vi "325 Read and Compressor auto control(SubVI).vi"(11 "Instrument":T2={"335 Resource"="", "Input (0:A)"=0, "Instrument Type"=enum."PPMS", "quantum design"=refnum, "Heater Output (1:1)"=0, "semaphore"=refnum, "TCP master instance"=refnum, "335 Status"=refnum, "M24C Resource"="GPIB0::24::INSTR", "4G supply"="GPIB0::24::INSTR", "Temp Status 24C"=refnum, "Temp"=refnum, "9T信号"=refnum, "limit"={"Field limit"=0.0, "Field rate limit"=0.0, "Temp limit"=0.0, "Temp low limit"=0.0, "Temp rate limit "=0.0}, "4g supply status"=refnum, "vi路径"="", "325 Resource "="GPIB0::24::INSTR", "Input (0:A) 325"=0, "Input (1;B)"=1, "in-plane"="", "out-plane"="", "in-plane"=FALSE, "out-plane"=FALSE, "in plane 信号"=refnum, "pzt volt"=refnum, "Aborting"=refnum, "数据文件"=refnum, "warning"=refnum, "750 visa"="", "750 rotate"="", "335 Status 2"=refnum} {"Input (1;B)" items=["A", "B"]; "Input (0:A) 325" items=["A", "B"]; "Input (0:A)" items=["A", "B"]; "Heater Output (1:1)" items=["1"=1, "2"=2]}) -> (2 "325 Temp":dbl, 3 "簇":T6 {"Heater Range" items=["Off", "Low (On)", "Medium", "High"]; "Heater Range 2" items=["Off", "Low (On)", "Medium", "High"]; "?" items=["Unknow", "Stable", "Following Warm", "Following Cold", "Unfollowing"]})   [LabVIEW 2019, in "Get value.lvlib"]
uses:
  Get value.lvlib
  ctl/335 state.ctl
  ctl/Instrument.ctl
  <vilib>/NI/Modbus Library/API/Master/Modbus Master.lvclass
  ctl/Instrument Type.ctl
  lib/QDInstrument.dll
  ctl/limit.ctl
  ctl/9T mag field stauts.ctl
  ctl/warning.ctl
  lib/Lake Shore 335/Lake Shore 335.lvlib
panel:
  out "下拉列表":T1=2 items=["Unknow", "Stable", "Following Warm", "Following Cold", "Unfollowing"]
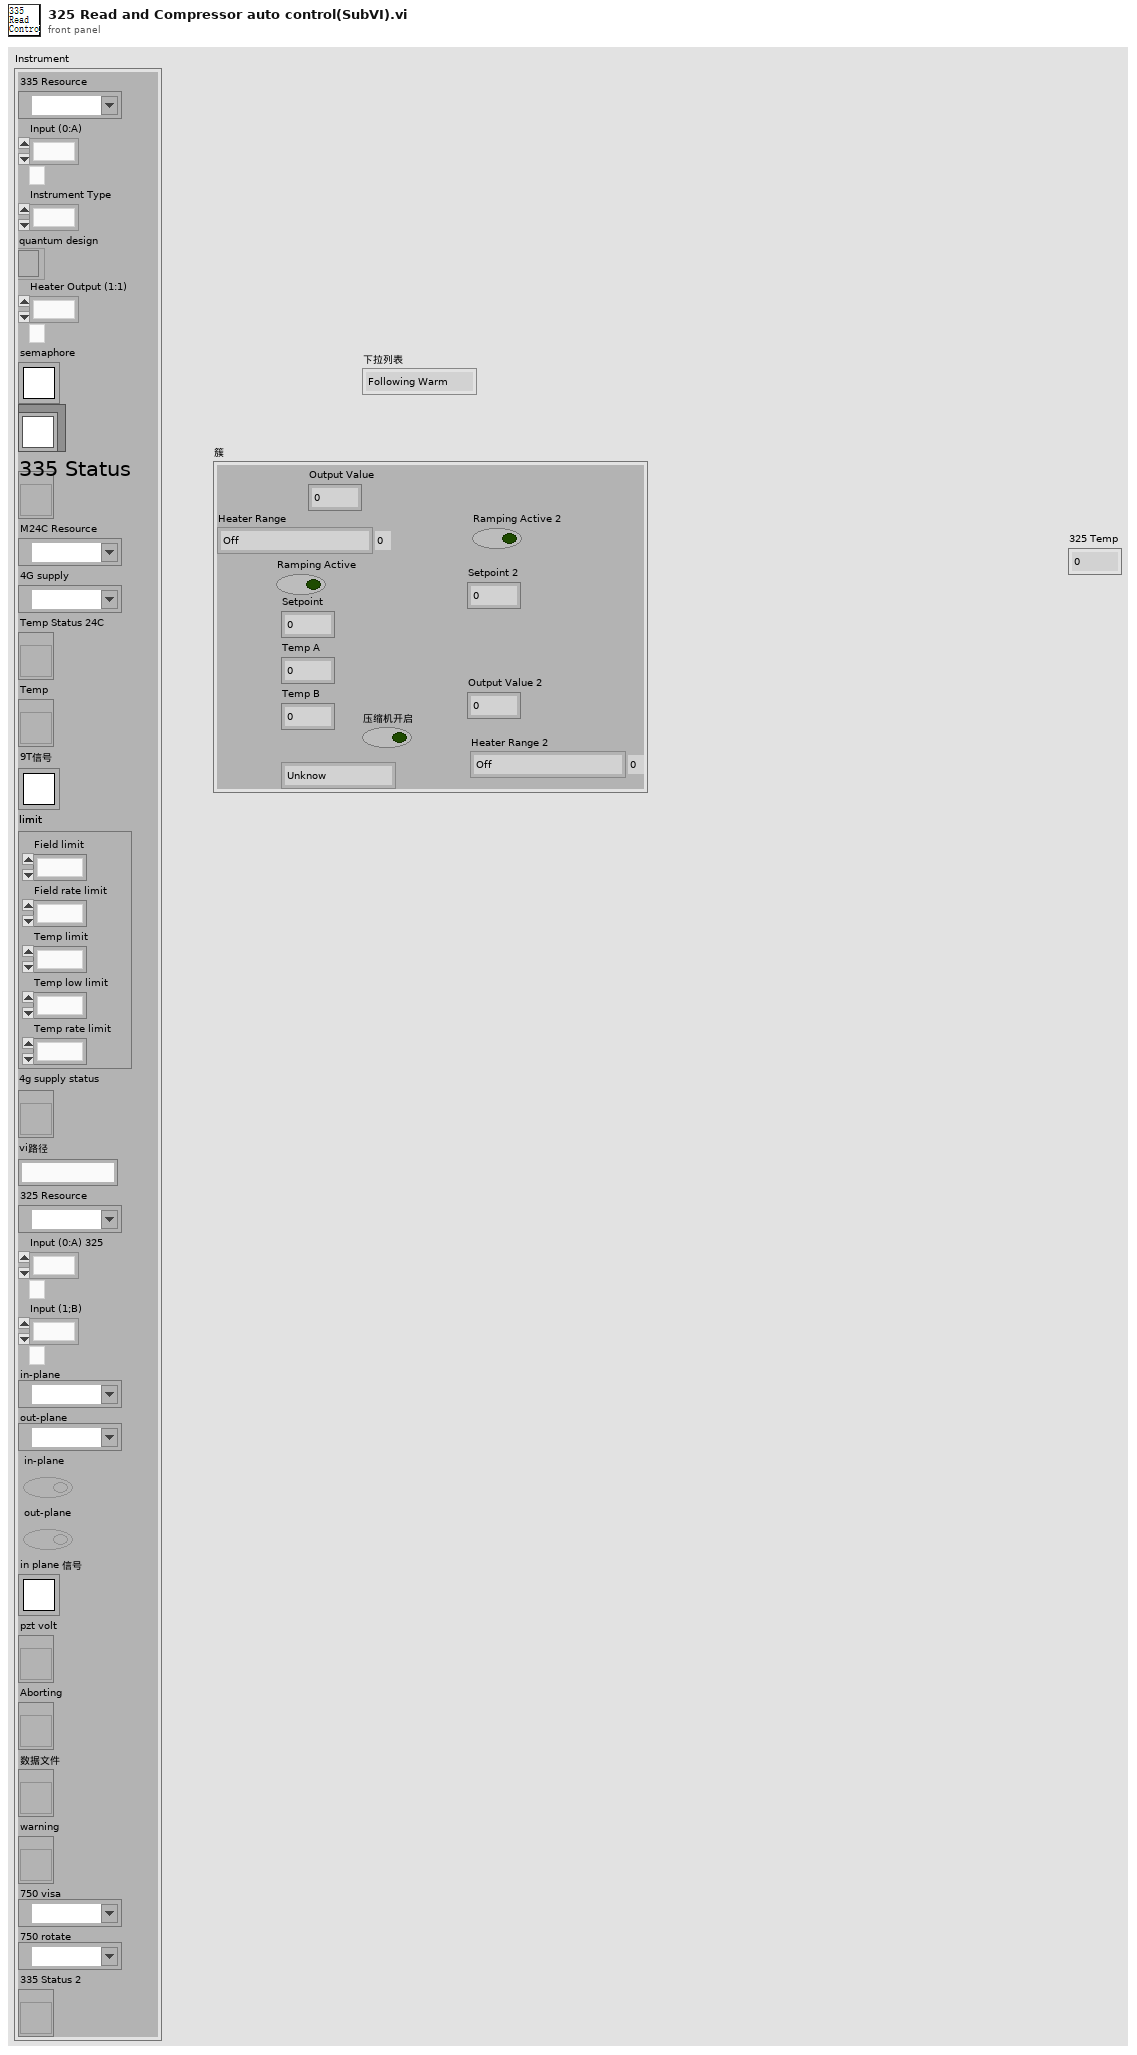
[diagram p1: front panel]
types:
  T1 = typedef "335 state.ctl" = u16
  T2 = typedef "Instrument.ctl" = cluster{"335 Resource":refnum<visa-resource-name>, "Input (0:A)":u16, "Instrument Type":T3, "quantum design":refnum<k24>, "Heater Output (1:1)":u16, "semaphore":T4, "TCP master instance":refnum<class "Modbus Master.lvclass">, "335 Status":refnum<vi>, "M24C Resource":refnum<visa-resource-name>, "4G supply":refnum<visa-resource-name>, "Temp Status 24C":refnum<vi>, "Temp":refnum<vi>, "9T信号":T4, "limit":T5, "4g supply status":refnum<vi>, "vi路径":string, "325 Resource ":refnum<visa-resource-name>, "Input (0:A) 325":u16, "Input (1;B)":u16, "in-plane":refnum<visa-resource-name>, "out-plane":refnum<visa-resource-name>, "in-plane":bool, "out-plane":bool, "in plane 信号":T4, "pzt volt":refnum<vi>, "Aborting":refnum<vi>, "数据文件":refnum<vi>, "warning":refnum<vi>, "750 visa":refnum<visa-resource-name>, "750 rotate":refnum<visa-resource-name>, "335 Status 2":refnum<vi>}
  T3 = typedef "Instrument Type.ctl" = enum16{"PPMS", "VersaLab", "DynaCool", "SVSM", "PPMS-Rotate", "Lakeshore335", "lengtou2", "9T mag", "9T cmag rotate", "test"}
  T4 = typedef "Semaphore RefNum" = refnum<k1>
  T5 = typedef "limit.ctl" = cluster{"Field limit":dbl, "Field rate limit":dbl, "Temp limit":dbl, "Temp low limit":dbl, "Temp rate limit ":dbl}
  T6 = cluster{"Output Value":dbl, "Heater Range":u16, "Ramping Active":bool, "Setpoint":dbl, "Temp A":dbl, "Temp B":dbl, "压缩机开启":bool, T1, "Ramping Active 2":bool, "Setpoint 2":dbl, "Output Value 2":dbl, "Heater Range 2":u16}
  T7 = cluster{"Output Value":dbl, "Heater Range ":u16, "Ramping Active":bool, "Setpoint":dbl, "Sensor Data":dbl, "Sensor Data":dbl, bool, T1, "Ramping Active":bool, "Setpoint":dbl, "Output Value":dbl, "Heater Range ":u16}
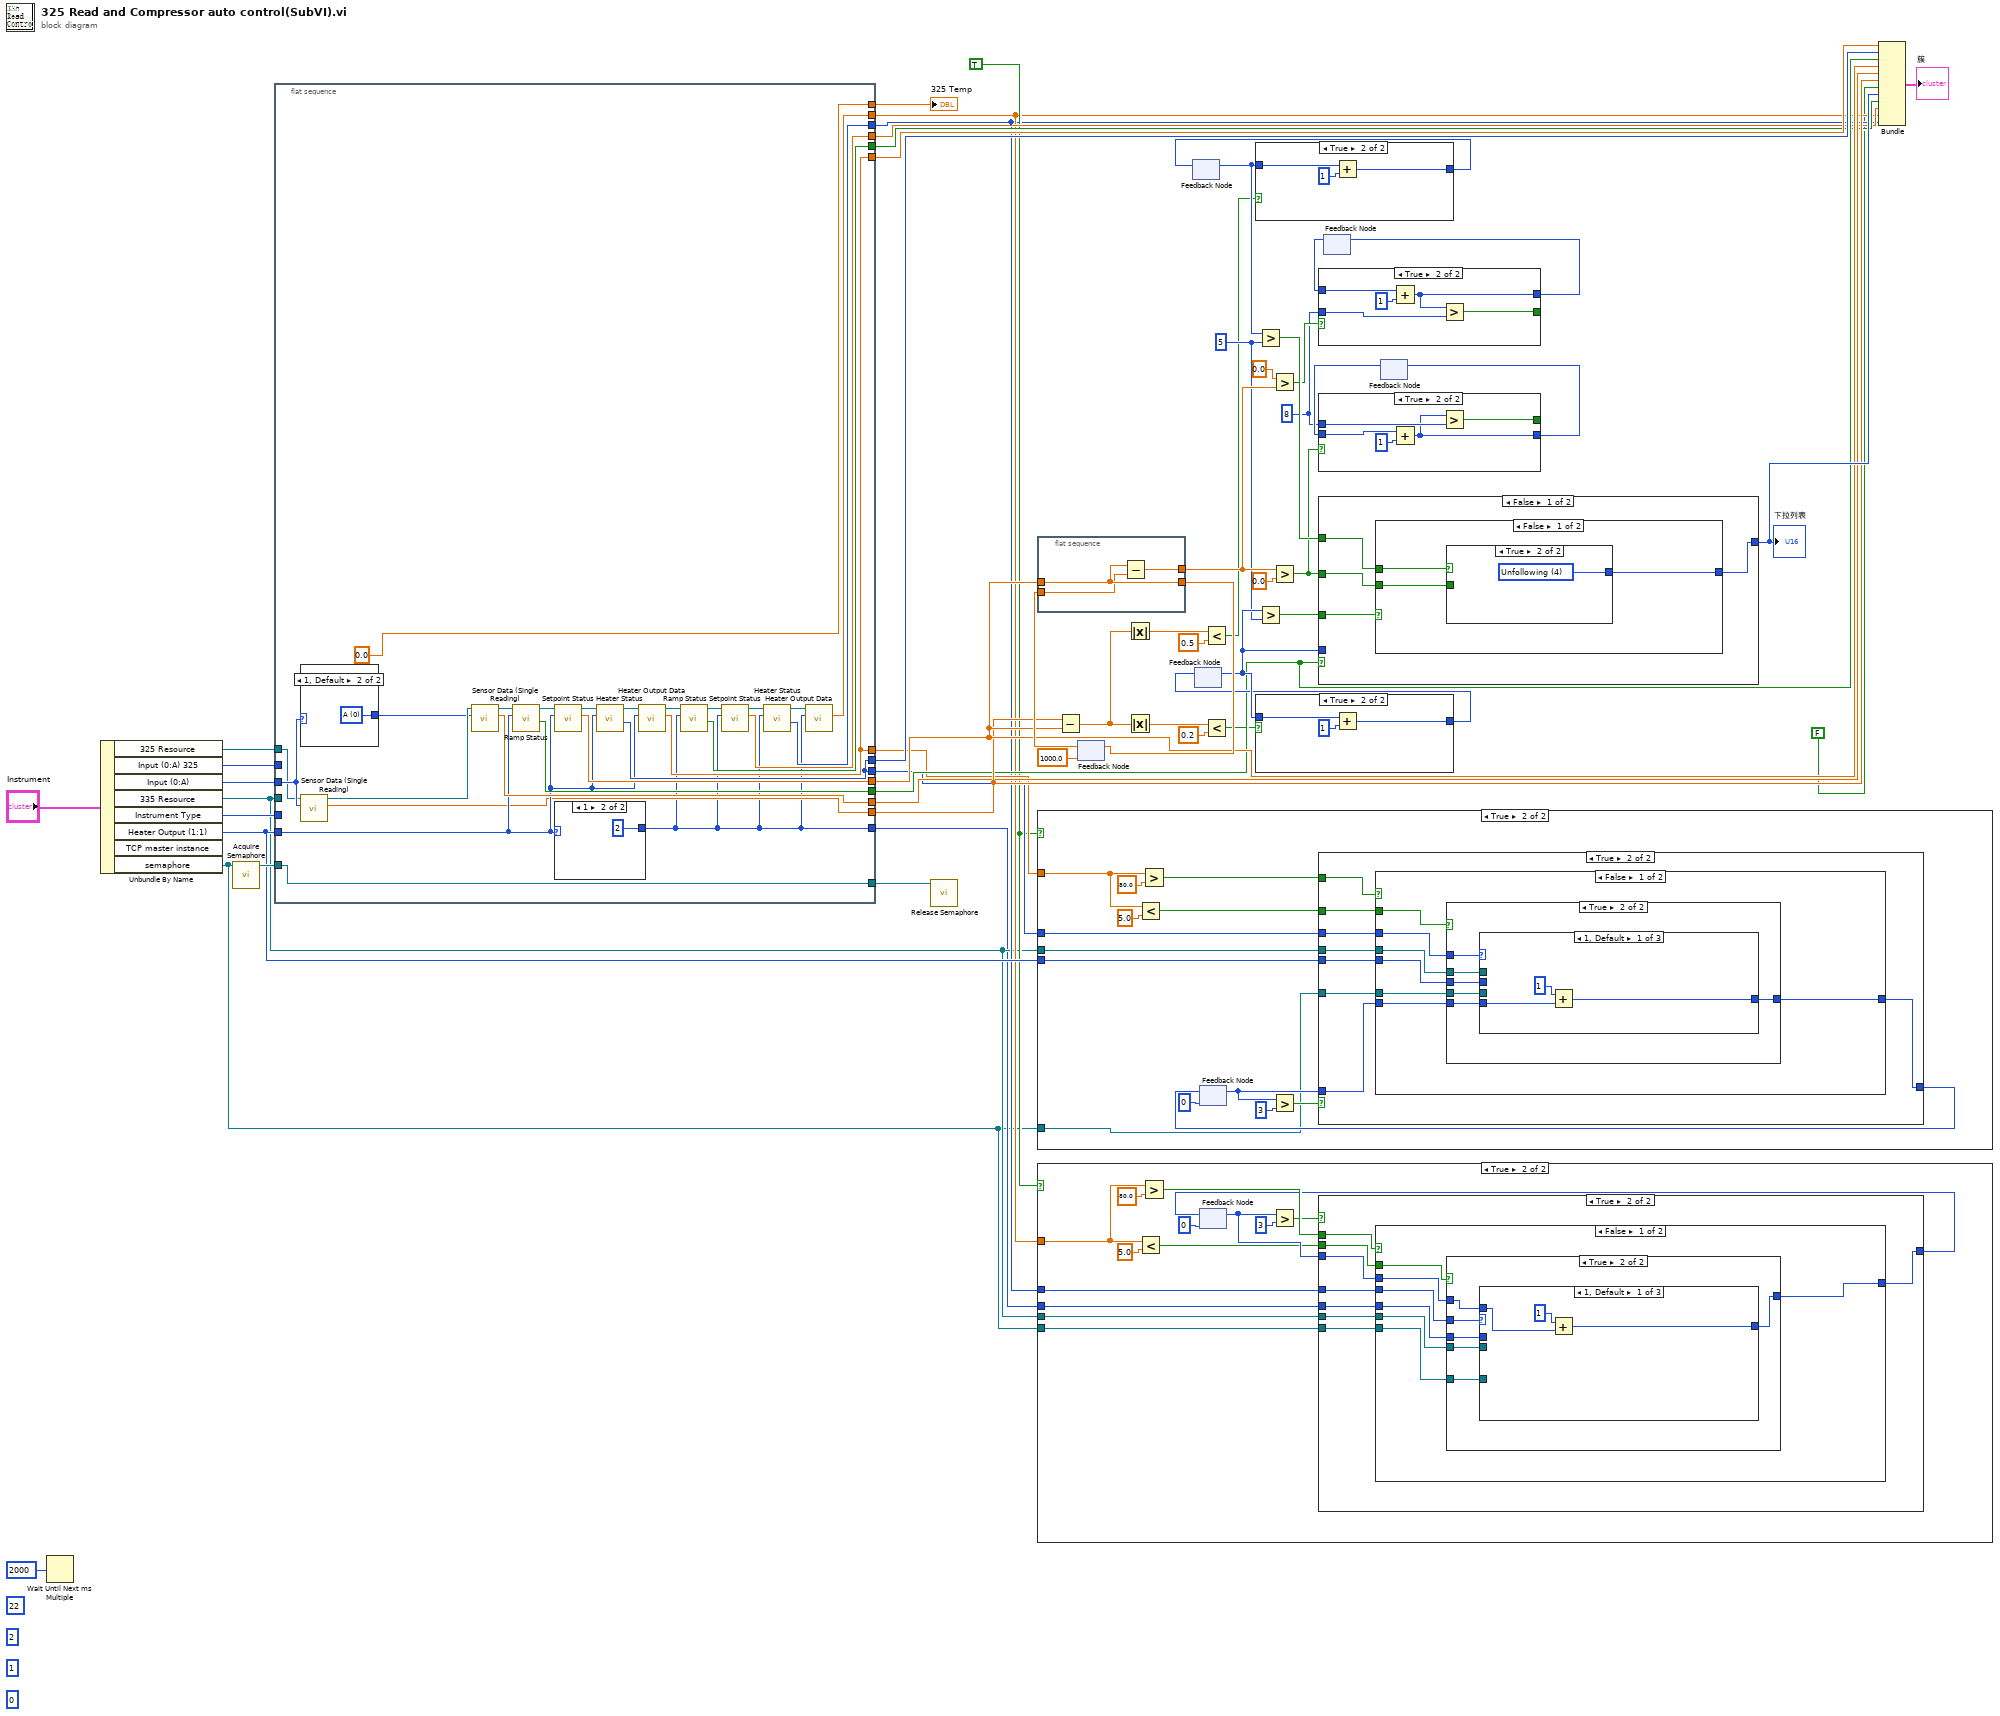
[diagram p0: block diagram]
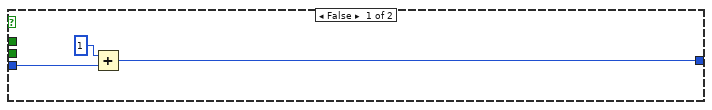
[diagram p3: hidden frame]
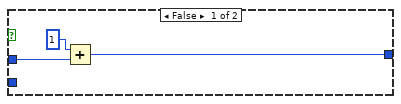
[diagram p4: hidden frame]
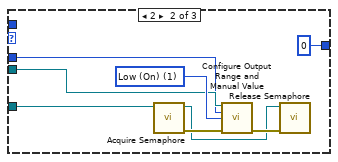
[diagram p5: hidden frame]
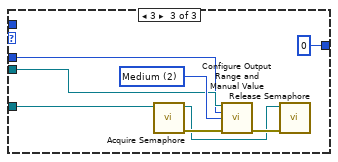
[diagram p6: hidden frame]
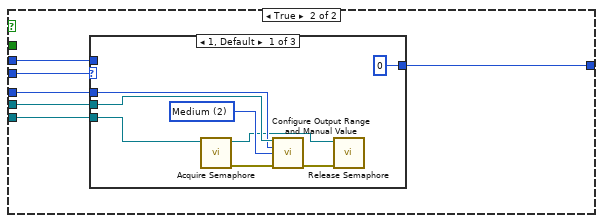
[diagram p7: hidden frame]
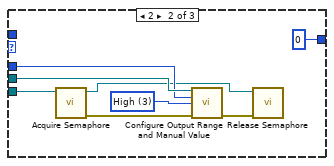
[diagram p8: hidden frame]
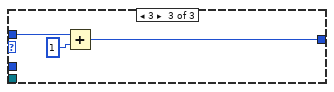
[diagram p9: hidden frame]
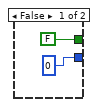
[diagram p10: hidden frame]
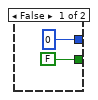
[diagram p11: hidden frame]
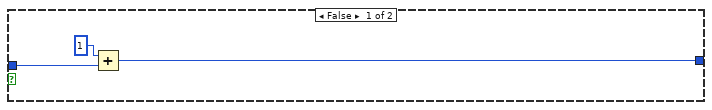
[diagram p13: hidden frame]
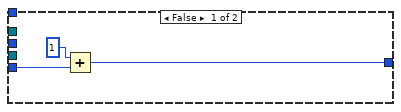
[diagram p14: hidden frame]
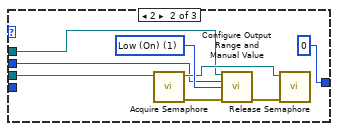
[diagram p15: hidden frame]
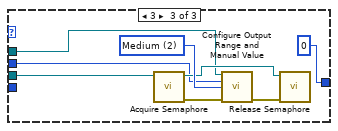
[diagram p16: hidden frame]
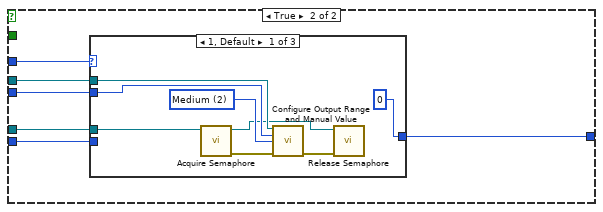
[diagram p17: hidden frame]
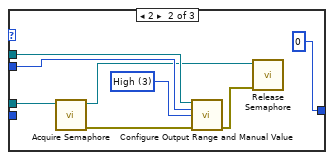
[diagram p18: hidden frame]
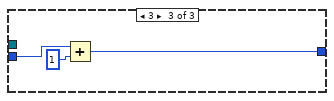
[diagram p19: hidden frame]
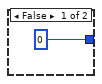
[diagram p20: hidden frame]
diagram:
  w14 = 8 ("y")
  w8 = TRUE
  w40 = 5 ("y")
  (unwired) 1 ("index")
  (unwired) 0 ("index")
  (unwired) u16 2 ("number of inputs")
  (unwired) u16 22 ("starting address")
  n1 = Wait Until Next ms Multiple(millisecond multiple=u32 2000) -> ()  [unwired: 1 out]
  n2 = Unbundle By Name("Instrument") -> ("325 Resource"=w13:refnum<visa-resource-name>, "Input (0:A) 325"=w12:u16, "Input (0:A)"=w28:u16, "335 Resource"=w5:refnum<visa-resource-name>, "Instrument Type"=w25:T3, "Heater Output (1:1)"=w21:u16, "semaphore"=w3:T4)  [unwired: 1 out]
  n3 = call <vilib>:"Acquire Semaphore.vi"("semaphore"=w3) -> ("semaphore out"=w26:T4)  [unwired: 4 in, 2 out]
  n4 = flat-sequence {
    tunnel: [w82] -> w49
    tunnel: w5 -> [_]
    tunnel: [w61] -> w44
    tunnel: w25 -> [_]
    tunnel: w26 -> [w78]
    tunnel: [w78] -> w27
    tunnel: [w72] -> w30
    tunnel: [w73] -> w29
    tunnel: [w77] -> w43
    tunnel: w21 -> [w66]
    tunnel: w28 -> [w60]
    tunnel: [w74] -> w31
    tunnel: [w73] -> w23
    tunnel: [w72] -> w22
    tunnel: w13 -> [w57]
    tunnel: w12 -> [_]
    tunnel: [0.0 ("Sensor Data")] -> w11
    tunnel: [w65] -> w10
    tunnel: [w64] -> w9
    tunnel: [w63] -> w6
    tunnel: [w62] -> w7
    tunnel: [w59] -> w4
    frame #0 {
      n5 = case shown="1, Default" w60 {
        tunnel: [w85 w86] -> w71
        frame 0 {
          w85 = u16 1 items=["A", "B"] ("Input (0:A)")
        }
        frame 1, Default {
          w86 = u16 0 items=["A", "B"] ("Input (0:A)")
        }
      }
      n6 = call "Sensor Data (Single Reading).vi"("Input (0:A)"=w60, "VISA resource name"=w57) -> ("Sensor Data"=w61:dbl, "VISA resource name out"=w76:refnum<visa-resource-name>)  [unwired: 7 in, 1 out]
      n7 = call "Sensor Data (Single Reading).vi"("Input (0:A)"=w71, "VISA resource name"=w76) -> ("Sensor Data"=w74:dbl, "VISA resource name out"=w75:refnum<visa-resource-name>)  [unwired: 7 in, 1 out]
      n8 = call "Ramp Status.vi"("Output's Control Loop (1:1)"=w66, "VISA resource name"=w75) -> ("Ramping Active"=w77:bool, "VISA resource name out"=w81:refnum<visa-resource-name>)  [unwired: 5 in, 3 out]
      n9 = call "Setpoint Status.vi"("Output (1:1)"=w66, "VISA resource name"=w81) -> ("Setpoint"=w82:dbl, "VISA resource name out"=w80:refnum<visa-resource-name>)  [unwired: 7 in, 1 out]
      n10 = case shown="1" w66 {
        tunnel: [1 2] -> w59
        frame 2, Default {
        }
        frame 1 {
        }
      }
      n11 = call "Heater Status.vi"("Heater Output (1:1)"=w66, "VISA resource name"=w80) -> ("Heater Range"=w72:u16, "VISA resource name out"=w79:refnum<visa-resource-name>)  [unwired: 5 in, 3 out]
      n12 = call "Heater Output Data.vi"("Heater Output (1:1)"=w66, "VISA resource name"=w79) -> ("Output Value"=w73:dbl, "VISA resource name out"=w70:refnum<visa-resource-name>)  [unwired: 7 in, 1 out]
      n13 = call "Ramp Status.vi"("Output's Control Loop (1:1)"=w59, "VISA resource name"=w70) -> ("Ramping Active"=w65:bool, "VISA resource name out"=w69:refnum<visa-resource-name>)  [unwired: 5 in, 3 out]
      n14 = call "Setpoint Status.vi"("Output (1:1)"=w59, "VISA resource name"=w69) -> ("Setpoint"=w64:dbl, "VISA resource name out"=w68:refnum<visa-resource-name>)  [unwired: 7 in, 1 out]
      n15 = call "Heater Status.vi"("Heater Output (1:1)"=w59, "VISA resource name"=w68) -> ("Heater Range"=w63:u16, "VISA resource name out"=w67:refnum<visa-resource-name>)  [unwired: 5 in, 3 out]
      n16 = call "Heater Output Data.vi"("Heater Output (1:1)"=w59, "VISA resource name"=w67) -> ("Output Value"=w62:dbl)  [unwired: 7 in, 2 out]
    }
  }
  n17 = call <vilib>:"Release Semaphore.vi"("semaphore"=w27) -> ()  [unwired: 5 in, 2 out]
  n18 = flat-sequence {
    tunnel: w49 -> [w89]
    tunnel: [w89] -> w50
    tunnel: w51 -> [w88]
    tunnel: [w87] -> w56
    frame #0 {
      n19 = Subtract(x=w89, y=w88) -> (x-y=w87:dbl)
    }
  }
  n20 = case shown="True" w8 {
    tunnel: w23 -> [_ w102]
    tunnel: w22 -> [_ w99]
    tunnel: w5 -> [_ w98]
    tunnel: w21 -> [_ w97]
    tunnel: w3 -> [_ w90]
    frame False {
    }
    frame True {
      n21 = Less?(x=w102, y=5.0) -> (x < y?=w92:bool)
      n22 = Greater?(x=w102, y=80.0) -> (0:w100:bool)
      n23 = feedback #1(0) -> (w93:i32)
      n24 = Greater?(x=w93, y=3) -> (0:w95:bool)
      n25 = case shown="True" w95 {
        tunnel: w100 -> [_ w114]
        tunnel: w99 -> [_ w113]
        tunnel: w98 -> [_ w112]
        tunnel: w97 -> [_ w111]
        tunnel: w90 -> [_ w110]
        tunnel: [w104 w109] -> w94
        tunnel: w93 -> [w106 w108]
        tunnel: w92 -> [_ w107]
        frame False {
          n26 = Add(x=1, y=w106) -> (x+y=w104:i32)
        }
        frame True {
          n27 = case shown="False" w114 {
            tunnel: w113 -> [w121 w155]
            tunnel: w112 -> [w120 w154]
            tunnel: w111 -> [w119 w153]
            tunnel: w110 -> [w116 w152]
            tunnel: [w118 w151] -> w109
            tunnel: w108 -> [w117 w150]
            tunnel: w107 -> [w115 _]
            frame False {
              n28 = case shown="True" w115 {
                tunnel: w121 -> [_ w130]
                tunnel: w120 -> [_ w129]
                tunnel: w119 -> [_ w128]
                tunnel: [w122 w127] -> w118
                tunnel: w117 -> [w124 w126]
                tunnel: w116 -> [_ w125]
                frame False {
                  n29 = Add(x=1, y=w124) -> (x+y=w122:i32)
                }
                frame True {
                  n30 = case shown="1, Default" w130 {
                    tunnel: w129 -> [_ w137 w145]
                    tunnel: w128 -> [_ w136 w144]
                    tunnel: [w131 0 0] -> w127
                    tunnel: w126 -> [w133 _ _]
                    tunnel: w125 -> [_ w134 w142]
                    frame 1, Default {
                      n31 = Add(x=1, y=w133) -> (x+y=w131:i32)
                    }
                    frame 2 {
                      w141 = u16 1 items=["Off", "Low (On)", "Medium", "High"] ("Range (0:Off)")
                      n32 = call <vilib>:"Acquire Semaphore.vi"("semaphore"=w134) -> ("error out"=w140:errorcluster, "semaphore out"=w138:T4)  [unwired: 4 in, 1 out]
                      n33 = call "Configure Output Range and Manual Value.vi"("VISA resource name"=w137, "Heater Output (1:1)"=w136, "Range (0:Off)"=w141, "error in (no error)"=w140) -> ("error out"=w139:errorcluster)  [unwired: 10 in, 1 out]
                      n34 = call <vilib>:"Release Semaphore.vi"("error in (no error)"=w139, "semaphore"=w138) -> ()  [unwired: 4 in, 2 out]
                    }
                    frame 3 {
                      w149 = u16 2 items=["Off", "Low (On)", "Medium", "High"] ("Range (0:Off)")
                      n35 = call <vilib>:"Acquire Semaphore.vi"("semaphore"=w142) -> ("error out"=w148:errorcluster, "semaphore out"=w146:T4)  [unwired: 4 in, 1 out]
                      n36 = call "Configure Output Range and Manual Value.vi"("VISA resource name"=w145, "Heater Output (1:1)"=w144, "Range (0:Off)"=w149, "error in (no error)"=w148) -> ("error out"=w147:errorcluster)  [unwired: 10 in, 1 out]
                      n37 = call <vilib>:"Release Semaphore.vi"("error in (no error)"=w147, "semaphore"=w146) -> ()  [unwired: 4 in, 2 out]
                    }
                  }
                }
              }
            }
            frame True {
              n38 = case shown="1, Default" w155 {
                tunnel: w154 -> [w163 w171 _]
                tunnel: w153 -> [w162 w170 _]
                tunnel: w152 -> [w156 w165 _]
                tunnel: [0 0 w172] -> w151
                tunnel: w150 -> [_ _ w174]
                frame 1, Default {
                  w159 = u16 2 items=["Off", "Low (On)", "Medium", "High"] ("Range (0:Off)")
                  n39 = call <vilib>:"Acquire Semaphore.vi"("semaphore"=w156) -> ("error out"=w160:errorcluster, "semaphore out"=w158:T4)  [unwired: 4 in, 1 out]
                  n40 = call "Configure Output Range and Manual Value.vi"("VISA resource name"=w163, "Heater Output (1:1)"=w162, "Range (0:Off)"=w159, "error in (no error)"=w160) -> ("error out"=w161:errorcluster)  [unwired: 10 in, 1 out]
                  n41 = call <vilib>:"Release Semaphore.vi"("error in (no error)"=w161, "semaphore"=w158) -> ()  [unwired: 4 in, 2 out]
                }
                frame 2 {
                  w169 = u16 3 items=["Off", "Low (On)", "Medium", "High"] ("Range (0:Off)")
                  n42 = call <vilib>:"Acquire Semaphore.vi"("semaphore"=w165) -> ("error out"=w168:errorcluster, "semaphore out"=w166:T4)  [unwired: 4 in, 1 out]
                  n43 = call "Configure Output Range and Manual Value.vi"("VISA resource name"=w171, "Heater Output (1:1)"=w170, "Range (0:Off)"=w169, "error in (no error)"=w168) -> ("error out"=w167:errorcluster)  [unwired: 10 in, 1 out]
                  n44 = call <vilib>:"Release Semaphore.vi"("error in (no error)"=w167, "semaphore"=w166) -> ()  [unwired: 4 in, 2 out]
                }
                frame 3 {
                  n45 = Add(x=w174, y=1) -> (x+y=w172:i32)
                }
              }
            }
          }
        }
      }
      n46 = feedback-in #1(w94) -> ()
    }
  }
  n47 = case shown="True" w8 {
    tunnel: w7 -> [_ w187]
    tunnel: w6 -> [_ w184]
    tunnel: w5 -> [_ w183]
    tunnel: w4 -> [_ w182]
    tunnel: w3 -> [_ w181]
    frame False {
    }
    frame True {
      n48 = Less?(x=w187, y=5.0) -> (x < y?=w176:bool)
      n49 = Greater?(x=w187, y=80.0) -> (0:w185:bool)
      n50 = feedback #2(0) -> (w177:i32)
      n51 = Greater?(x=w177, y=3) -> (0:w179:bool)
      n52 = case shown="True" w179 {
        tunnel: w185 -> [_ w199]
        tunnel: w184 -> [_ w198]
        tunnel: w183 -> [_ w197]
        tunnel: w182 -> [_ w196]
        tunnel: w181 -> [_ w195]
        tunnel: [w189 w194] -> w178
        tunnel: w177 -> [w191 w193]
        tunnel: w176 -> [_ w192]
        frame False {
          n53 = Add(x=1, y=w191) -> (x+y=w189:i32)
        }
        frame True {
          n54 = case shown="False" w199 {
            tunnel: w198 -> [w206 w240]
            tunnel: w197 -> [w205 w239]
            tunnel: w196 -> [w204 w238]
            tunnel: w195 -> [w201 w237]
            tunnel: [w203 w236] -> w194
            tunnel: w193 -> [w202 w235]
            tunnel: w192 -> [w200 _]
            frame False {
              n55 = case shown="True" w200 {
                tunnel: w206 -> [_ w215]
                tunnel: w205 -> [_ w214]
                tunnel: w204 -> [_ w213]
                tunnel: [w207 w212] -> w203
                tunnel: w202 -> [w209 w211]
                tunnel: w201 -> [_ w210]
                frame False {
                  n56 = Add(x=1, y=w209) -> (x+y=w207:i32)
                }
                frame True {
                  n57 = case shown="1, Default" w215 {
                    tunnel: w214 -> [_ w222 w230]
                    tunnel: w213 -> [_ w221 w229]
                    tunnel: [w216 0 0] -> w212
                    tunnel: w211 -> [w218 _ _]
                    tunnel: w210 -> [_ w219 w227]
                    frame 1, Default {
                      n58 = Add(x=1, y=w218) -> (x+y=w216:i32)
                    }
                    frame 2 {
                      w226 = u16 1 items=["Off", "Low (On)", "Medium", "High"] ("Range (0:Off)")
                      n59 = call <vilib>:"Acquire Semaphore.vi"("semaphore"=w219) -> ("error out"=w225:errorcluster, "semaphore out"=w223:T4)  [unwired: 4 in, 1 out]
                      n60 = call "Configure Output Range and Manual Value.vi"("VISA resource name"=w222, "Heater Output (1:1)"=w221, "Range (0:Off)"=w226, "error in (no error)"=w225) -> ("error out"=w224:errorcluster)  [unwired: 10 in, 1 out]
                      n61 = call <vilib>:"Release Semaphore.vi"("error in (no error)"=w224, "semaphore"=w223) -> ()  [unwired: 4 in, 2 out]
                    }
                    frame 3 {
                      w234 = u16 2 items=["Off", "Low (On)", "Medium", "High"] ("Range (0:Off)")
                      n62 = call <vilib>:"Acquire Semaphore.vi"("semaphore"=w227) -> ("error out"=w233:errorcluster, "semaphore out"=w231:T4)  [unwired: 4 in, 1 out]
                      n63 = call "Configure Output Range and Manual Value.vi"("VISA resource name"=w230, "Heater Output (1:1)"=w229, "Range (0:Off)"=w234, "error in (no error)"=w233) -> ("error out"=w232:errorcluster)  [unwired: 10 in, 1 out]
                      n64 = call <vilib>:"Release Semaphore.vi"("error in (no error)"=w232, "semaphore"=w231) -> ()  [unwired: 4 in, 2 out]
                    }
                  }
                }
              }
            }
            frame True {
              n65 = case shown="1, Default" w240 {
                tunnel: w239 -> [w248 w256 _]
                tunnel: w238 -> [w247 w255 _]
                tunnel: w237 -> [w241 w250 _]
                tunnel: [0 0 w257] -> w236
                tunnel: w235 -> [_ _ w259]
                frame 1, Default {
                  w244 = u16 2 items=["Off", "Low (On)", "Medium", "High"] ("Range (0:Off)")
                  n66 = call <vilib>:"Acquire Semaphore.vi"("semaphore"=w241) -> ("error out"=w245:errorcluster, "semaphore out"=w243:T4)  [unwired: 4 in, 1 out]
                  n67 = call "Configure Output Range and Manual Value.vi"("VISA resource name"=w248, "Heater Output (1:1)"=w247, "Range (0:Off)"=w244, "error in (no error)"=w245) -> ("error out"=w246:errorcluster)  [unwired: 10 in, 1 out]
                  n68 = call <vilib>:"Release Semaphore.vi"("error in (no error)"=w246, "semaphore"=w243) -> ()  [unwired: 4 in, 2 out]
                }
                frame 2 {
                  w254 = u16 3 items=["Off", "Low (On)", "Medium", "High"] ("Range (0:Off)")
                  n69 = call <vilib>:"Acquire Semaphore.vi"("semaphore"=w250) -> ("error out"=w253:errorcluster, "semaphore out"=w251:T4)  [unwired: 4 in, 1 out]
                  n70 = call "Configure Output Range and Manual Value.vi"("VISA resource name"=w256, "Heater Output (1:1)"=w255, "Range (0:Off)"=w254, "error in (no error)"=w253) -> ("error out"=w252:errorcluster)  [unwired: 10 in, 1 out]
                  n71 = call <vilib>:"Release Semaphore.vi"("error in (no error)"=w252, "semaphore"=w251) -> ()  [unwired: 4 in, 2 out]
                }
                frame 3 {
                  n72 = Add(x=w259, y=1) -> (x+y=w257:i32)
                }
              }
            }
          }
        }
      }
      n73 = feedback-in #2(w178) -> ()
    }
  }
  n74 = Subtract(x=w44, y=w49) -> (x-y=w38:dbl)
  n75 = feedback #3(1000.0 ("Setpoint")) -> (w51:dbl)
  n76 = feedback-in #3(w50) -> ()
  n77 = Absolute Value(x=w38) -> (abs(x)=w36:dbl)
  n78 = Absolute Value(x=w38) -> (abs(x)=w35:dbl)
  n79 = feedback #4() -> (w46:i32)  [unwired: 1 in]
  n80 = feedback #5() -> (w48:i32)  [unwired: 1 in]
  n81 = Less?(x=w36, y=0.5) -> (x < y?=w39:bool)
  n82 = Less?(x=w35, y=0.2) -> (x < y?=w34:bool)
  n83 = case shown="True" w39 {
    tunnel: w46 -> [_ w263]
    tunnel: [0 w261] -> w45
    frame False {
    }
    frame True {
      n84 = Add(x=w263, y=1) -> (x+y=w261:i32)
    }
  }
  n85 = feedback-in #4(w45) -> ()
  n86 = case shown="True" w34 {
    tunnel: w48 -> [_ w267]
    tunnel: [0 w265] -> w47
    frame False {
    }
    frame True {
      n87 = Add(x=w267, y=1) -> (x+y=w265:i32)
    }
  }
  n88 = feedback-in #5(w47) -> ()
  n89 = Greater?(x=w46, y=w40) -> (0:w42:bool)
  n90 = Greater?(x=w48, y=w40) -> (0:w41:bool)
  n91 = Greater?(x=0.0, y=w56) -> (0:w20:bool)
  n92 = Greater?(x=w56, y=0.0) -> (0:w15:bool)
  n93 = case shown="False" w43 {
    tunnel: w48 -> [_ _]
    tunnel: w41 -> [w271 _]
    tunnel: w42 -> [w270 w280]
    tunnel: [w269 w279] -> w54
    tunnel: w15 -> [w268 w278]
    frame False {
      n94 = case shown="False" w271 {
        tunnel: [w273 w277] -> w269
        tunnel: w270 -> [w274 _]
        tunnel: w268 -> [w272 _]
        frame False {
          n95 = case shown="True" w274 {
            tunnel: [w275 w276] -> w273
            tunnel: w272 -> [_ _]
            frame False {
              w275 = T1 4 items=["Unknow", "Stable", "Following Warm", "Following Cold", "Unfollowing"]
            }
            frame True {
              w276 = T1 4 items=["Unknow", "Stable", "Following Warm", "Following Cold", "Unfollowing"]
            }
          }
        }
        frame True {
          w277 = T1 1 items=["Unknow", "Stable", "Following Warm", "Following Cold", "Unfollowing"]
        }
      }
    }
    frame True {
      n96 = case shown="False" w280 {
        tunnel: [w281 w282] -> w279
        tunnel: w278 -> [_ w283]
        frame False {
          w281 = T1 4 items=["Unknow", "Stable", "Following Warm", "Following Cold", "Unfollowing"]
        }
        frame True {
          n97 = case shown="True" w283 {
            tunnel: [w284 w285] -> w282
            frame False {
              w284 = T1 3 items=["Unknow", "Stable", "Following Warm", "Following Cold", "Unfollowing"]
            }
            frame True {
              w285 = T1 2 items=["Unknow", "Stable", "Following Warm", "Following Cold", "Unfollowing"]
            }
          }
        }
      }
    }
  }
  "下拉列表" <- w54
  n98 = feedback #6() -> (w18:i32)  [unwired: 1 in]
  n99 = case shown="True" w20 {
    tunnel: [0 w290] -> w19
    tunnel: w18 -> [_ w291]
    tunnel: w14 -> [_ w289]
    tunnel: [FALSE w288] -> _
    frame False {
    }
    frame True {
      n100 = Add(x=w291, y=1) -> (x+y=w290:i32)
      n101 = Greater?(x=w290, y=w289) -> (0:w288:bool)
    }
  }
  n102 = feedback-in #6(w19) -> ()
  n103 = feedback #7() -> (w17:i32)  [unwired: 1 in]
  n104 = case shown="True" w15 {
    tunnel: [0 w296] -> w16
    tunnel: w17 -> [_ w298]
    tunnel: w14 -> [_ w297]
    tunnel: [FALSE w295] -> _
    frame False {
    }
    frame True {
      n105 = Add(x=w298, y=1) -> (x+y=w296:i32)
      n106 = Greater?(x=w296, y=w297) -> (0:w295:bool)
    }
  }
  n107 = feedback-in #7(w16) -> ()
  n108 = Bundle("Output Value"=w29, "Heater Range"=w30, "Ramping Active"=w43, "Setpoint"=w49, "Sensor Data"=w31, "Sensor Data"=w44, FALSE, w54, "Ramping Active"=w10, "Setpoint"=w9, "Output Value"=w7, "Heater Range"=w6) -> (→"簇":T7)  [unwired: 1 in]
  "325 Temp" <- w11
